vi "prependLength.vi"(5 "msg in":string) -> (2 "msg out":string)   [LabVIEW 2015]
doc: "Prepends the length of the string."
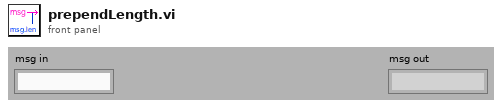
[diagram p1: front panel]
types:
  T1 = enum16{"big-endian, network order", "native, host order", "little-endian"}
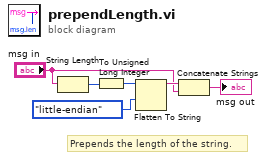
[diagram p0: block diagram]
diagram:
  # "Prepends the length of the string."
  n1 = String Length(string="msg in") -> (length=w4:i32)
  n2 = To Unsigned Long Integer(number=w4) -> (unsigned 32bit integer=w3:u32)
  n3 = Flatten To String(anything=w3, byte order (0:big-endian, network order)=T1."little-endian") -> (data string=w6:string)  [unwired: 2 in, 2 out]
  n4 = Concatenate Strings(w6, "msg in") -> (→"msg out":string)
